vi "Measure.vi"(8 "error in (no error)":errorcluster, 11 "Diode IV in":refnum<class "Diode IV.lvclass">) -> (0 "error out":errorcluster, 3 "Diode IV out":refnum<class "Diode IV.lvclass">)   [LabVIEW 2015, in "Diode Characterization.lvlib" / "Diode IV.lvclass"]
uses:
  Diode IV.lvclass
  Results/I-V Report/I-V Result.lvclass
  <userlib>/Common Components/Measurement Actor/Measurement.lvclass/Measurement.ctl
  <userlib>/Common Components/Measurement Actor/Measurement.lvclass
  <userlib>/Common Components/Results/Results.lvclass
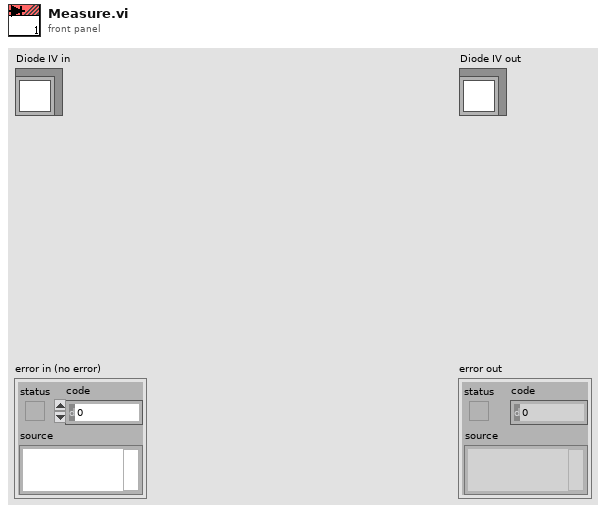
[diagram p1: front panel]
types:
  T1 = typedef "Diode Characterization.lvlib/Diode IV.lvclass/graphdata.ctl" = cluster{"Data":waveform(dbl)[], "AnntList":T2, "CrsrList":T3, "Analysis Data":waveform(dbl)[]}
  T2 = typedef "LVAnnotationListTypeDef.ctl" = cluster{"Name":string, "Color":u32, "Style":u8, "Point Style":u8, "Name Visible":bool, "Allow Drag":bool, "Annotation Mode":u32, "Plot":i32, "Index":i32, "Position":cluster{"X":dbl, "Y":dbl}, "X Scale":u32, "Y Scale":u32, "Show Arrow":bool, "Lock Name":bool, "Plot Area":i32, "Label Offset":cluster{"X":dbl, "Y":dbl}}[]
  T3 = typedef "LVCursorListTypeDef.ctl" = cluster{"Name":string, "Color":u32, "Style":u8, "Point Style":u8, "Name Visible":bool, "Allow Drag":bool, "Cursor Mode":u32, "Plot":i32, "Index":i32, "Position":cluster{"X":dbl, "Y":dbl}, "X Scale":u32, "Y Scale":u32, "Watch Plots":i32[], "Watch All Plots":bool, "Plot Area":i32, "Label Offset":cluster{"X":dbl, "Y":dbl}}[]
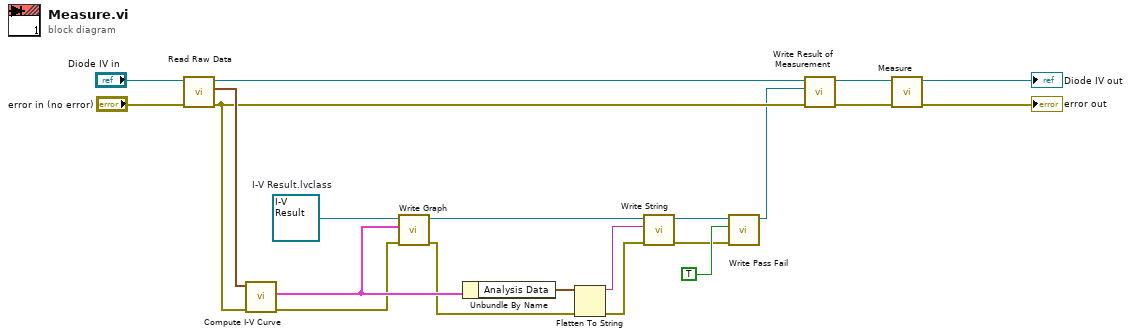
[diagram p0: block diagram]
diagram:
  w15 = refnum<class "I-V Result.lvclass"> refnum  # I-V Result.lvclass
  n1 = call "Read Raw Data.vi"("error in (no error)"="error in (no error)", "Diode I-V in"="Diode IV in") -> ("error out"=w10:errorcluster, "Raw Data"=w11:waveform(dbl), "Diode I-V out"=w21:refnum<class "Diode IV.lvclass">)  [unwired: 7 in]
  n2 = call "Compute I-V Curve.vi"("error in (no error)"=w10, "Waveform"=w11) -> ("error out"=w7:errorcluster, "Merged Graph Data"=w13:T1)  [unwired: 8 in]
  n3 = call "Write Graph.vi"("error in (no error)"=w7, "Graph"=w13, "I-V Result in"=w15) -> ("error out"=w8:errorcluster, "I-V Result out"=w14:refnum<class "I-V Result.lvclass">)  [unwired: 7 in]
  n4 = Unbundle By Name(w13) -> ("Analysis Data"=w19:waveform(dbl)[])
  n5 = Flatten To String(anything=w19, error in (no error)=w8) -> (data string=w18:string, error out=w6:errorcluster)  [unwired: 2 in, 1 out]
  n6 = call <userlib>:"Write String.vi"("error in (no error)"=w6, "String"=w18, "Results in"=w14) -> ("error out"=w9:errorcluster, "Results out"=w20:refnum<class "I-V Result.lvclass">)  [unwired: 7 in]
  n7 = call <userlib>:"Write Pass Fail.vi"("error in (no error)"=w9, "Pass Fail"=TRUE, "Results in"=w20) -> ("Results out"=w5:refnum<class "I-V Result.lvclass">)  [unwired: 7 in, 1 out]
  n8 = call <userlib>:"Write Result of Measurement.vi"("error in (no error)"=w10, "Result Actor.lvlib:Results.lvclass"=w5, "Measurement in"=w21) -> ("error out"=w3:errorcluster, "Measurement out"=w4:refnum<class "Diode IV.lvclass">)  [unwired: 7 in]
  n9 = call-parent "Measure.vi"("error in (no error)"=w3, "Measurement in"=w4) -> ("error out"=→"error out":errorcluster, "Measurement out"=→"Diode IV out":refnum<class "Diode IV.lvclass">)  [unwired: 8 in]
